vi "Send Message.vi"(8 "error in":errorcluster, 11 "Message in":refnum<class "Message.lvclass">) -> (0 "error out":errorcluster, 3 "Message out":refnum<class "Message.lvclass">)   [LabVIEW 2014, in "Message.lvclass"]
uses:
  Message.lvclass
  Topic_class/Topic.lvclass
  Message.lvclass/Message.ctl
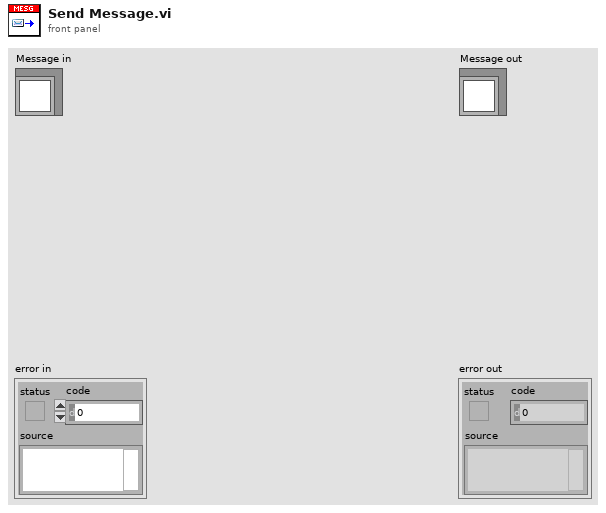
[diagram p1: front panel]
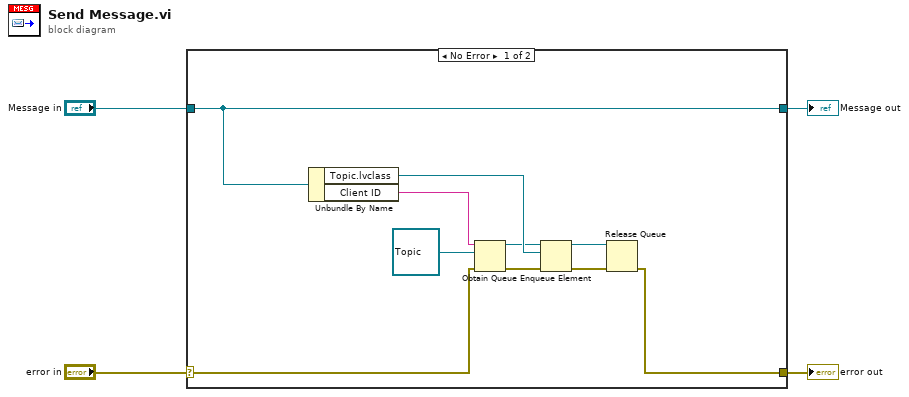
[diagram p0: block diagram]
diagram:
  n1 = case shown="No Error" "error in" {
    selector: "error in" -> [w6 w16]
    tunnel: [w5 w16] -> w3
    tunnel: [w14 w15] -> w1
    tunnel: "Message in" -> [w14 w15]
    frame No Error {
      n2 = Unbundle By Name(w14) -> ("Topic.lvclass"=w11:refnum<class "Topic.lvclass">, "Client ID"=w12:string)
      n3 = Obtain Queue(name (unnamed)=w12, element data type=refnum<class "Topic.lvclass"> refnum ("Topic.lvclass"), error in (no error)=w6) -> (queue out=w10:refnum<queue>, error out=w8:errorcluster)  [unwired: 2 in, 1 out]
      n4 = Enqueue Element(queue=w10, element=w11, error in (no error)=w8) -> (queue out=w9:refnum<queue>, error out=w7:errorcluster)  [unwired: 1 in, 1 out]
      n5 = Release Queue(queue=w9, error in (no error)=w7) -> (error out=w5:errorcluster)  [unwired: 1 in, 2 out]
    }
    frame Error {
    }
  }
  "error out" <- w3
  "Message out" <- w1
